vi "Discrete Integrator (DBL).vi"(2 "initialize":bool, 3 "initial condition":dbl format="%.2f", 5 "input point":dbl format="%.2f") -> (1 "output point":dbl format="%.2f")   [LabVIEW 2017, in "NI_AdvCtrl_discrete linear.lvlib"]
doc: "LabVIEW no longer supports this VI. You can obtain similar functionality by installing the LabVIEW Simulation Module.\n\nIntegrates a discrete input signal. The integration process is based on Euler method."
uses:
  <vilib>/addons/control/advanced/NI_AdvCtrl_discrete linear.lvlib
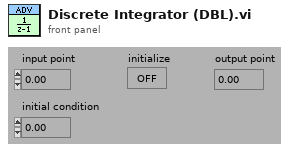
[diagram p1: front panel]
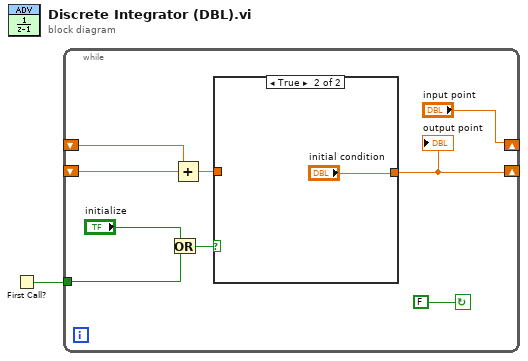
[diagram p0: block diagram]
diagram:
  n1 = First Call?() -> (First Call?: T/F=w1:bool)
  n2 = while {
    shift-left: _ -> [w2]
    shift-right: ["input point"] -> _
    tunnel: w1 -> [w7]
    shift-left: _ -> [w5]
    shift-right: [w10] -> _
    stop <- FALSE continue-if-true
    n3 = Or(x="initialize", y=w7) -> (x .or. y?=w6:bool)
    n4 = Add(x=w2, y=w5) -> (x+y=w4:dbl)
    n5 = case shown="True" w6 {
      tunnel: [w11 "initial condition"] -> w10
      tunnel: w4 -> [w11 _]
      frame False {
      }
      frame True {
      }
    }
    "output point" <- w10
  }
